vi "报告存储.vi"(8 "生成报告?":bool, 9 "是否存储到数据库?":bool, 11 "试验时间":timestamp) -> ()   [LabVIEW 2010]
uses:
  <vilib>/Utility/NIReport.llb/NI_report.lvclass
  全局量/试验配置信息.vi
  全局量/自动测试结果.vi
  <vilib>/Utility/NIReport.llb/Append Report Text (str wrap).vi
  全局量/全局_配置.vi
  <vilib>/addons/_office/word.llb/Word Easy Table (str).vi
  <vilib>/addons/_office/NI_ReportGenerationToolkit.lvlib
panel:
  in  "序号 2":i32
  in  "序号":i32
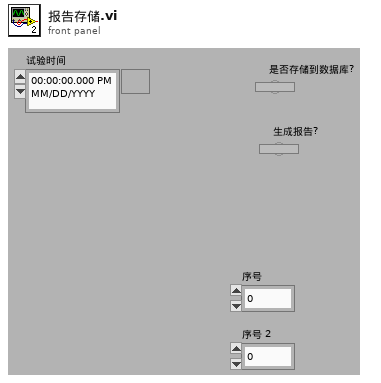
[diagram p1: front panel]
types:
  T1 = enum16{"maximized", "minimized", "normal", "no change"}
  T2 = enum16{"Standard Report", "HTML", "Word", "Excel"}
  T3 = cluster{"position (Excel)":cluster{"row":i32, "column":i32}, "name (Excel)":string, "bookmark (Word)":string}
  T4 = cluster{"报告编号":string, "控制板编号":string, "控制板类型":string, "测试人员":string, "测试地点":string, string, u64, "spreadsheet string":string, "spreadsheet string":string, "spreadsheet string":string, "spreadsheet string":string, "格式字符串":string}
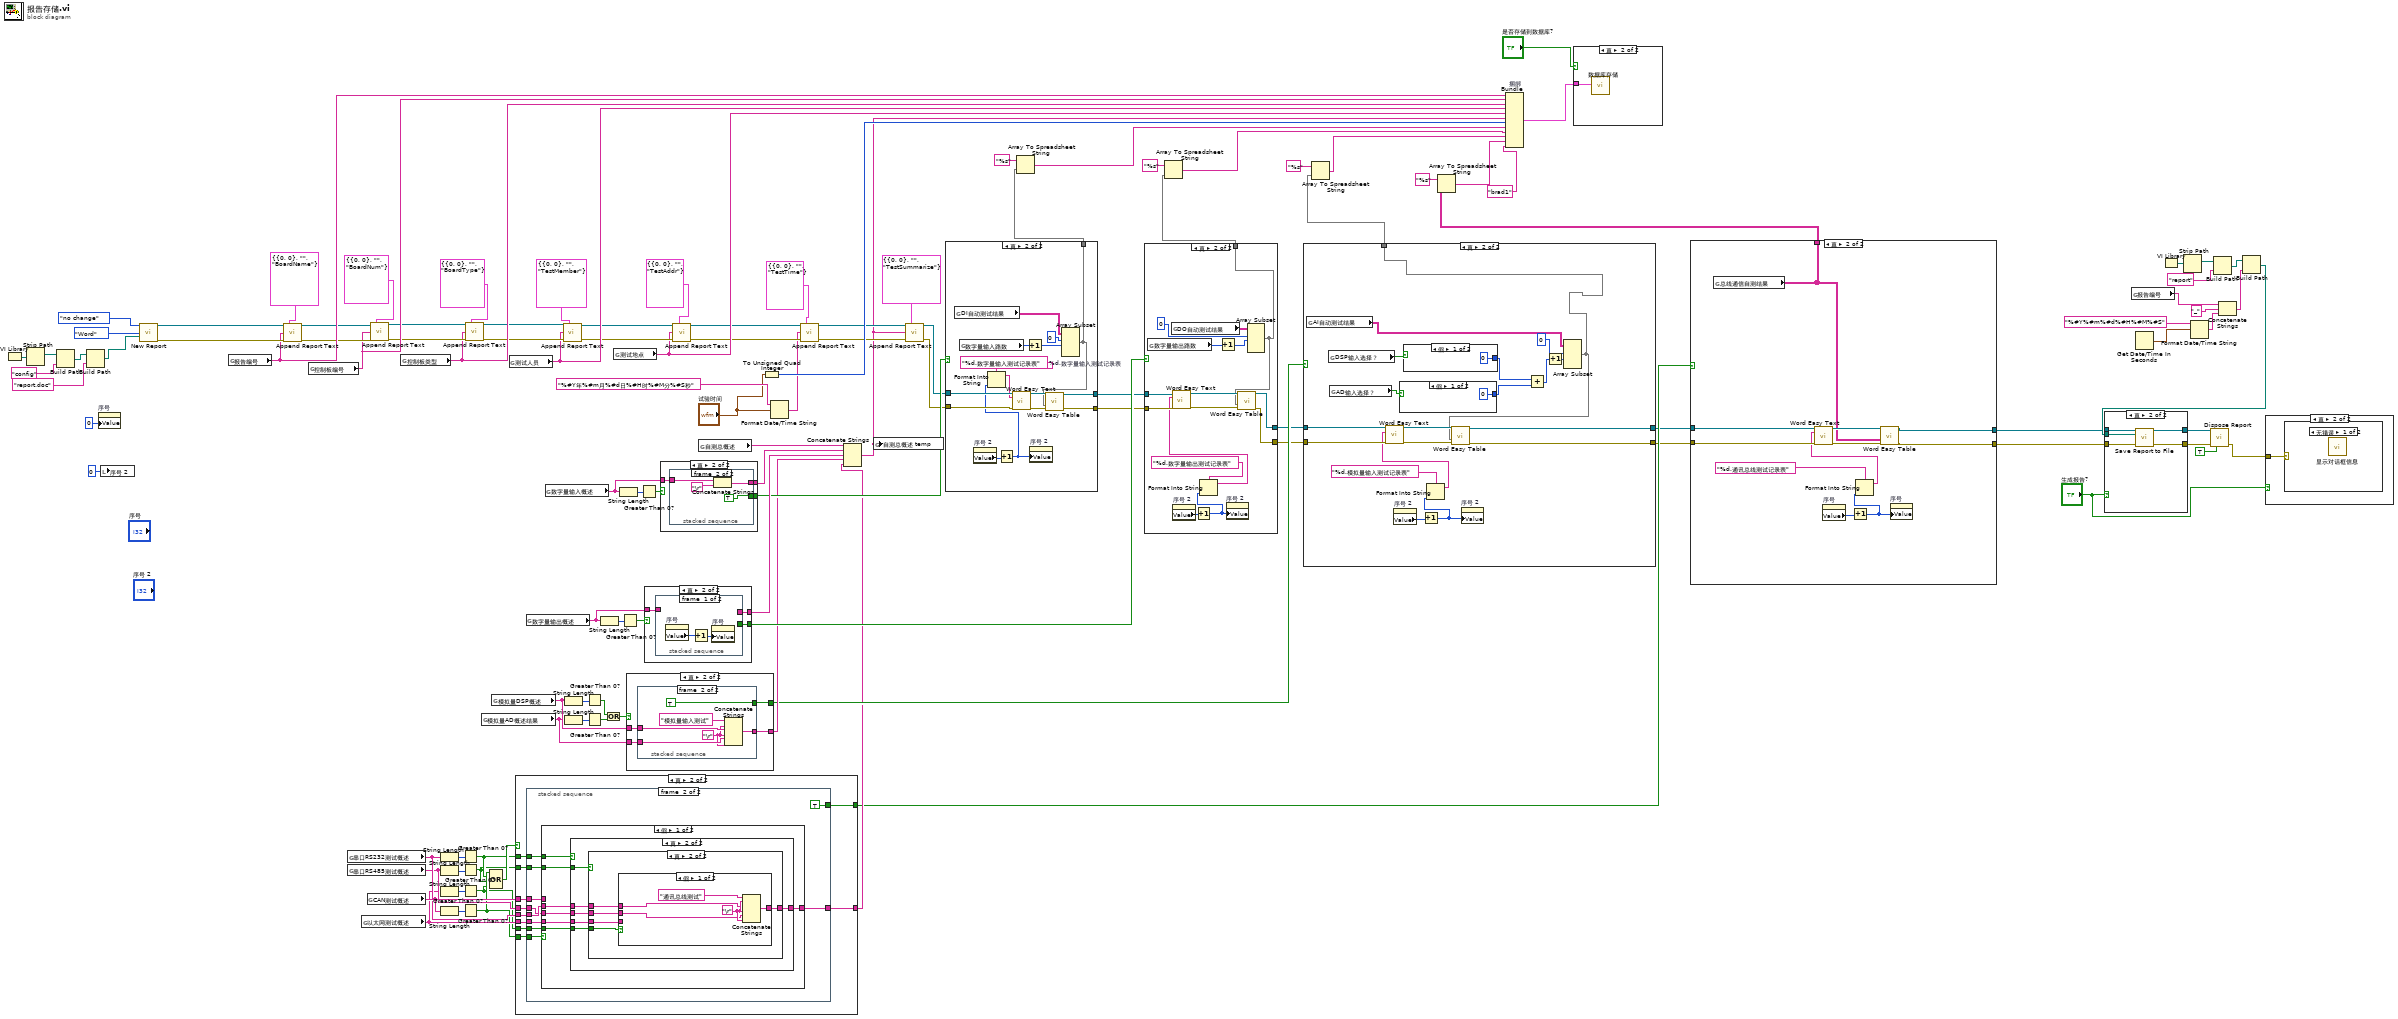
[diagram p0: block diagram]
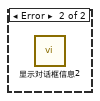
[diagram p3: hidden frame]
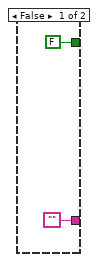
[diagram p6: hidden frame]
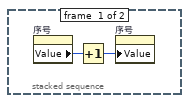
[diagram p7: hidden frame]
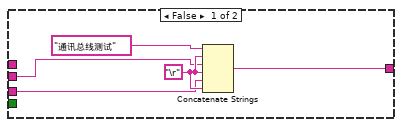
[diagram p8: hidden frame]
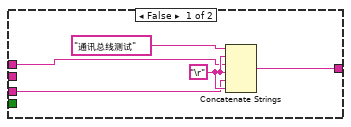
[diagram p9: hidden frame]
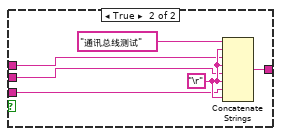
[diagram p10: hidden frame]
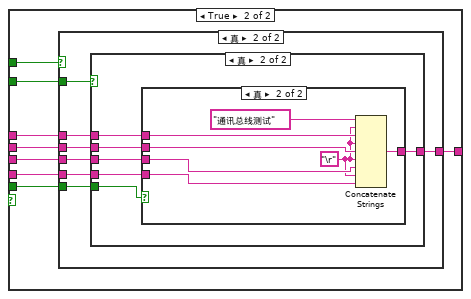
[diagram p11: hidden frame]
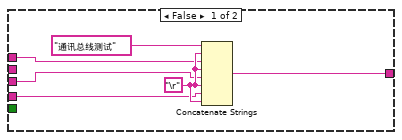
[diagram p12: hidden frame]
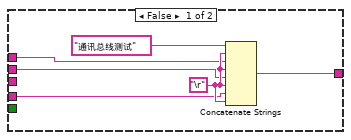
[diagram p13: hidden frame]
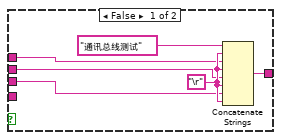
[diagram p14: hidden frame]
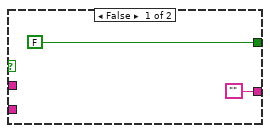
[diagram p15: hidden frame]
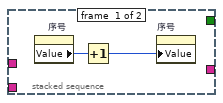
[diagram p16: hidden frame]
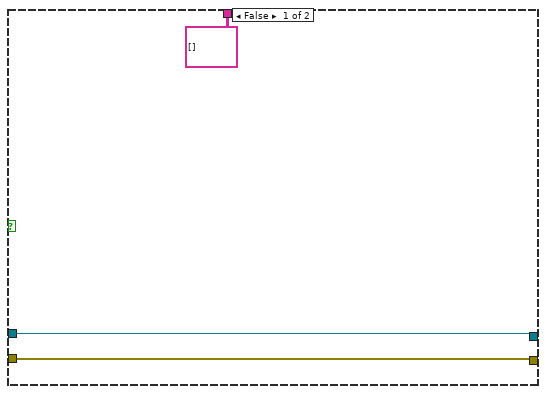
[diagram p17: hidden frame]
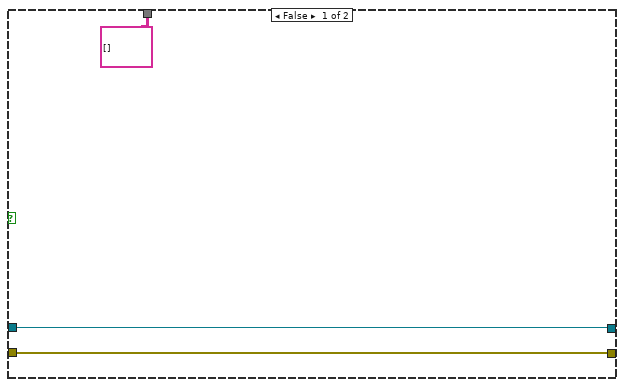
[diagram p18: hidden frame]
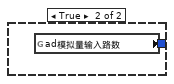
[diagram p19: hidden frame]
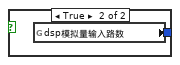
[diagram p20: hidden frame]
diagram:
  n1 = VI Library() -> (path=w67:path)
  n2 = Strip Path(path=w67) -> (stripped path=w64:path)  [unwired: 1 out]
  n3 = Build Path(base path=w64, name or relative path="config") -> (appended path=w66:path)
  n4 = Build Path(base path=w66, name or relative path="report.doc") -> (appended path=w70:path)
  n5 = property on="序号" class="DigNum (严格)"("Value"=0 ("序号")) -> ()  [unwired: 2 in, 2 out]
  n6 = local write "序号 2"(0 ("序号 2")) -> ()
  n7 = call <vilib>:"New Report.vi"("window state (normal)"=T1."no change", "report type"=T2."Word", "template (empty)"=w70) -> ("report out"=w62:refnum<class "NI_report.lvclass">, "error out"=w61:errorcluster)  [unwired: 11 in]
  n8 = global read "试验配置信息.vi" "报告编号"() -> (w60:string)
  n9 = call-poly <vilib>:"Append Report Text.vi"("report in"=w62, "MS Office parameters"=T3 {"position (Excel)"={"row"=0, "column"=0}, "name (Excel)"="", "bookmark (Word)"="BoardName"}, "text"=w60, "error in (no error)"=w61) -> ("report out"=w58:refnum<class "NI_report.lvclass">, "error out"=w57:errorcluster)  [unwired: 8 in, 2 out]
  n10 = global read "试验配置信息.vi" "控制板编号"() -> (w56:string)
  n11 = global read "自动测试结果.vi" "串口RS232测试概述"() -> (w76:string)
  n12 = global read "自动测试结果.vi" "串口RS485测试概述"() -> (w75:string)
  n13 = global read "自动测试结果.vi" "以太网测试概述"() -> (w74:string)
  n14 = global read "自动测试结果.vi" "CAN测试概述"() -> (w77:string)
  n15 = call-poly <vilib>:"Append Report Text.vi"("report in"=w58, "MS Office parameters"=T3 {"position (Excel)"={"row"=0, "column"=0}, "name (Excel)"="", "bookmark (Word)"="BoardNum"}, "text"=w56, "error in (no error)"=w57) -> ("report out"=w54:refnum<class "NI_report.lvclass">, "error out"=w53:errorcluster)  [unwired: 8 in, 2 out]
  n16 = global read "试验配置信息.vi" "控制板类型"() -> (w52:string)
  n17 = String Length(string=w76) -> (length=w80:i32)
  n18 = String Length(string=w75) -> (length=w81:i32)
  n19 = String Length(string=w74) -> (length=w82:i32)
  n20 = String Length(string=w77) -> (length=w79:i32)
  n21 = Greater Than 0?(x=w80) -> (x > 0?=w4:bool)
  n22 = Greater Than 0?(x=w81) -> (x > 0?=w3:bool)
  n23 = Greater Than 0?(x=w82) -> (x > 0?=w2:bool)
  n24 = Greater Than 0?(x=w79) -> (x > 0?=w5:bool)
  n25 = call-poly <vilib>:"Append Report Text.vi"("report in"=w54, "MS Office parameters"=T3 {"position (Excel)"={"row"=0, "column"=0}, "name (Excel)"="", "bookmark (Word)"="BoardType"}, "text"=w52, "error in (no error)"=w53) -> ("report out"=w50:refnum<class "NI_report.lvclass">, "error out"=w49:errorcluster)  [unwired: 8 in, 2 out]
  n26 = global read "自动测试结果.vi" "模拟量AD概述结果"() -> (w85:string)
  n27 = Compound Arithmetic op=OR(w5, w4, w3, w2) -> (w78:bool)
  n28 = global read "自动测试结果.vi" "模拟量DSP概述"() -> (w86:string)
  n29 = global read "试验配置信息.vi" "测试人员"() -> (w48:string)
  n30 = case shown="真" w78 {
    tunnel: ["" w125] -> w73
    tunnel: [FALSE w124] -> w72
    tunnel: w77 -> [_ w129]
    tunnel: w76 -> [_ w128]
    tunnel: w75 -> [_ w127]
    tunnel: w74 -> [_ w126]
    tunnel: w5 -> [_ w123]
    tunnel: w4 -> [_ w122]
    tunnel: w3 -> [_ w121]
    tunnel: w2 -> [_ w120]
    frame False {
    }
    frame True {
      n31 = stacked-sequence {
        tunnel: w129 -> [_ w141]
        tunnel: w128 -> [_ w140]
        tunnel: w127 -> [_ w139]
        tunnel: w126 -> [_ w138]
        tunnel: [_ w137] -> w125
        tunnel: [_ TRUE] -> w124
        tunnel: w123 -> [_ w135]
        tunnel: w122 -> [_ w134]
        tunnel: w121 -> [_ w133]
        tunnel: w120 -> [_ w132]
        frame #0 {
          n32 = property on="序号" class="DigNum (严格)"() -> ("Value"=w130:i32)  [unwired: 2 in, 2 out]
          n33 = Increment(x=w130) -> (x+1=w131:i32)
          n34 = property on="序号" class="DigNum (严格)"("Value"=w131) -> ()  [unwired: 2 in, 2 out]
        }
        frame #1 {
          n35 = case shown="假" w135 {
            tunnel: w141 -> [_ w188]
            tunnel: w140 -> [w147 w187]
            tunnel: w139 -> [w146 w186]
            tunnel: w138 -> [w145 w185]
            tunnel: [w148 w184] -> w137
            tunnel: w134 -> [w144 w183]
            tunnel: w133 -> [w143 w182]
            tunnel: w132 -> [w142 w181]
            frame False {
              n36 = case shown="真" w144 {
                tunnel: [w149 w159] -> w148
                tunnel: w147 -> [_ w158]
                tunnel: w146 -> [w151 w157]
                tunnel: w145 -> [w150 w156]
                tunnel: w143 -> [_ w155]
                tunnel: w142 -> [_ w154]
                frame False {
                  w152 = "\r"
                  n37 = Concatenate Strings("通讯总线测试", w152, w151, w152, w150, w152) -> (w149:string)
                }
                frame True {
                  n38 = case shown="真" w155 {
                    tunnel: [w162 w169] -> w159
                    tunnel: w158 -> [w161 w168]
                    tunnel: w157 -> [_ w167]
                    tunnel: w156 -> [w160 w166]
                    tunnel: w154 -> [_ w165]
                    frame False {
                      w163 = "\r"
                      n39 = Concatenate Strings("通讯总线测试", w163, w161, w163, w160, w163) -> (w162:string)
                    }
                    frame True {
                      n40 = case shown="假" w165 {
                        tunnel: [w172 w178] -> w169
                        tunnel: w168 -> [w171 w177]
                        tunnel: w167 -> [w170 w176]
                        tunnel: w166 -> [_ w175]
                        frame False {
                          w173 = "\r"
                          n41 = Concatenate Strings("通讯总线测试", w173, w171, w173, w170, w173) -> (w172:string)
                        }
                        frame True {
                          w179 = "\r"
                          n42 = Concatenate Strings("通讯总线测试", w179, w177, w179, w176, w179, w175, w179) -> (w178:string)
                        }
                      }
                    }
                  }
                }
              }
            }
            frame True {
              n43 = case shown="真" w183 {
                tunnel: w188 -> [w191 w201]
                tunnel: w187 -> [_ w200]
                tunnel: w186 -> [w190 w199]
                tunnel: w185 -> [w189 w198]
                tunnel: [w192 w197] -> w184
                tunnel: w182 -> [_ w196]
                tunnel: w181 -> [_ w195]
                frame False {
                  w194 = "\r"
                  n44 = Concatenate Strings("通讯总线测试", w194, w191, w194, w190, w194, w189, w194) -> (w192:string)
                }
                frame True {
                  n45 = case shown="真" w196 {
                    tunnel: w201 -> [w204 w213]
                    tunnel: w200 -> [w203 w212]
                    tunnel: w199 -> [_ w211]
                    tunnel: w198 -> [w202 w210]
                    tunnel: [w205 w209] -> w197
                    tunnel: w195 -> [_ w208]
                    frame False {
                      w206 = "\r"
                      n46 = Concatenate Strings("通讯总线测试", w206, w204, w206, w203, w206, w202, w206) -> (w205:string)
                    }
                    frame True {
                      n47 = case shown="真" w208 {
                        tunnel: w213 -> [w216 w225]
                        tunnel: w212 -> [w215 w224]
                        tunnel: w211 -> [w214 w223]
                        tunnel: w210 -> [_ w222]
                        tunnel: [w218 w220] -> w209
                        frame False {
                          w217 = "\r"
                          n48 = Concatenate Strings("通讯总线测试", w217, w216, w217, w215, w217, w214, w217) -> (w218:string)
                        }
                        frame True {
                          w221 = "\r"
                          n49 = Concatenate Strings("通讯总线测试", w221, w225, w221, w224, w221, w223, w221, w222) -> (w220:string)
                        }
                      }
                    }
                  }
                }
              }
            }
          }
        }
      }
    }
  }
  n50 = global read "自动测试结果.vi" "数字量输出概述"() -> (w114:string)
  n51 = global read "自动测试结果.vi" "数字量输入概述"() -> (w115:string)
  n52 = call-poly <vilib>:"Append Report Text.vi"("report in"=w50, "MS Office parameters"=T3 {"position (Excel)"={"row"=0, "column"=0}, "name (Excel)"="", "bookmark (Word)"="TestMember"}, "text"=w48, "error in (no error)"=w49) -> ("report out"=w45:refnum<class "NI_report.lvclass">, "error out"=w44:errorcluster)  [unwired: 8 in, 2 out]
  n53 = String Length(string=w86) -> (length=w90:i32)
  n54 = String Length(string=w85) -> (length=w88:i32)
  n55 = Greater Than 0?(x=w90) -> (x > 0?=w89:bool)
  n56 = Greater Than 0?(x=w88) -> (x > 0?=w87:bool)
  n57 = String Length(string=w114) -> (length=w112:i32)
  n58 = Or(x=w89, y=w87) -> (x .or. y?=w91:bool)
  n59 = global read "试验配置信息.vi" "测试地点"() -> (w43:string)
  n60 = String Length(string=w115) -> (length=w117:i32)
  n61 = Greater Than 0?(x=w112) -> (x > 0?=w113:bool)
  n62 = case shown="真" w91 {
    tunnel: ["" w230] -> w84
    tunnel: w86 -> [_ w232]
    tunnel: w85 -> [_ w231]
    tunnel: [FALSE w229] -> w83
    frame False {
    }
    frame True {
      n63 = stacked-sequence {
        tunnel: w232 -> [_ w240]
        tunnel: w231 -> [_ w239]
        tunnel: [_ w238] -> w230
        tunnel: [_ TRUE] -> w229
        frame #0 {
          n64 = property on="序号" class="DigNum (严格)"() -> ("Value"=w234:i32)  [unwired: 2 in, 2 out]
          n65 = Increment(x=w234) -> (x+1=w233:i32)
          n66 = property on="序号" class="DigNum (严格)"("Value"=w233) -> ()  [unwired: 2 in, 2 out]
        }
        frame #1 {
          w236 = "\r"
          n67 = Concatenate Strings("模拟量输入测试", w236, w240, w236, w239, w236) -> (w238:string)
        }
      }
    }
  }
  n68 = Greater Than 0?(x=w117) -> (x > 0?=w116:bool)
  n69 = case shown="真" w113 {
    tunnel: w114 -> [_ w245]
    tunnel: ["" w244] -> w109
    tunnel: [FALSE w243] -> w106
    frame False {
    }
    frame True {
      n70 = stacked-sequence {
        tunnel: w245 -> [_ w251]
        tunnel: [_ w249] -> w244
        tunnel: [_ TRUE] -> w243
        frame #0 {
          n71 = property on="序号" class="DigNum (严格)"() -> ("Value"=w247:i32)  [unwired: 2 in, 2 out]
          n72 = Increment(x=w247) -> (x+1=w246:i32)
          n73 = property on="序号" class="DigNum (严格)"("Value"=w246) -> ()  [unwired: 2 in, 2 out]
        }
        frame #1 {
          n74 = Concatenate Strings(w251, "\r") -> (w249:string)
        }
      }
    }
  }
  n75 = case shown="真" w116 {
    tunnel: w115 -> [_ w256]
    tunnel: ["" w255] -> w110
    tunnel: [FALSE w254] -> w107
    frame False {
    }
    frame True {
      n76 = stacked-sequence {
        tunnel: w256 -> [_ w262]
        tunnel: [_ w260] -> w255
        tunnel: [_ TRUE] -> w254
        frame #0 {
          n77 = property on="序号" class="DigNum (严格)"() -> ("Value"=w257:i32)  [unwired: 2 in, 2 out]
          n78 = Increment(x=w257) -> (x+1=w258:i32)
          n79 = property on="序号" class="DigNum (严格)"("Value"=w258) -> ()  [unwired: 2 in, 2 out]
        }
        frame #1 {
          n80 = Concatenate Strings(w262, "\r") -> (w260:string)
        }
      }
    }
  }
  n81 = call-poly <vilib>:"Append Report Text.vi"("report in"=w45, "MS Office parameters"=T3 {"position (Excel)"={"row"=0, "column"=0}, "name (Excel)"="", "bookmark (Word)"="TestAddr"}, "text"=w43, "error in (no error)"=w44) -> ("report out"=w41:refnum<class "NI_report.lvclass">, "error out"=w40:errorcluster)  [unwired: 8 in, 2 out]
  n82 = global read "自动测试结果.vi" "自测总概述"() -> (w111:string)
  n83 = To Unsigned Quad Integer(1:"试验时间") -> (0:w105:u64)
  n84 = Format Date/Time String(time format string (%c)="%#Y年%#m月%#d日%#H时%#M分%#S秒" ("时间格式字符串(%c)"), seconds (now)="试验时间") -> (date/time string=w37:string)  [unwired: 1 in]
  n85 = call-poly <vilib>:"Append Report Text.vi"("report in"=w41, "MS Office parameters"=T3 {"position (Excel)"={"row"=0, "column"=0}, "name (Excel)"="", "bookmark (Word)"="TestTime"}, "text"=w37, "error in (no error)"=w40) -> ("report out"=w36:refnum<class "NI_report.lvclass">, "error out"=w35:errorcluster)  [unwired: 8 in, 2 out]
  n86 = Concatenate Strings(w111, w110, w109, w84, w73) -> (w33:string)
  n87 = global write "自动测试结果.vi" "自测总概述 temp"(w33) -> ()
  n88 = call-poly <vilib>:"Append Report Text.vi"("report in"=w36, "MS Office parameters"=T3 {"position (Excel)"={"row"=0, "column"=0}, "name (Excel)"="", "bookmark (Word)"="TestSummarize"}, "text"=w33, "error in (no error)"=w35) -> ("report out"=w32:refnum<class "NI_report.lvclass">, "error out"=w31:errorcluster)  [unwired: 8 in, 2 out]
  n89 = case shown="真" w107 {
    tunnel: [string[][] [] ("DI自动测试结果") w270] -> w103
    tunnel: w32 -> [w264 w276]
    tunnel: w31 -> [w263 w275]
    tunnel: [w264 w267] -> w30
    tunnel: [w263 w266] -> w29
    frame False {
    }
    frame True {
      w272 = "%d.数字量输入测试记录表"  # %d.数字量输入测试记录表
      n90 = global read "自动测试结果.vi" "DI自动测试结果"() -> (w279:string[][])
      n91 = global read "全局_配置.vi" "数字量输入路数"() -> (w278:i32)
      n92 = property on="序号 2" class="DigNum (严格)"() -> ("Value"=w269:i32)  [unwired: 2 in, 2 out]
      n93 = Increment(x=w269) -> (x+1=w268:i32)
      n94 = Format Into String(format string=w272, w268) -> (resulting string=w271:string)  [unwired: 2 in, 1 out]
      n95 = call <vilib>:"Word Easy Text.vi"("report in"=w276, "text"=w271, "error in (no error)"=w275) -> ("report out"=w274:refnum<class "NI_report.lvclass">, "error out"=w273:errorcluster)  [unwired: 10 in, 1 out]
      n96 = Increment(x=w278) -> (x+1=w277:i32)
      n97 = property on="序号 2" class="DigNum (严格)"("Value"=w268) -> ()  [unwired: 2 in, 2 out]
      n98 = Array Subset(array=w279, index (row)=0 ("索引"), length (row)=w277) -> (w270:string[][])  [unwired: 2 in]
      n99 = call-poly <vilib>:"Word Easy Table.vi"("report in"=w274, "data"=w270, "error in (no error)"=w273) -> ("report out"=w267:refnum<class "NI_report.lvclass">, "error out"=w266:errorcluster)  [unwired: 10 in, 1 out]
    }
  }
  n100 = Array To Spreadsheet String(array=w103, 3:"%s" ("格式字符串")) -> (spreadsheet string=w102:string)  [unwired: 1 in]
  n101 = case shown="真" w106 {
    tunnel: [string[][] [] ("DO自动测试结果") w286] -> w100
    tunnel: w30 -> [w282 w291]
    tunnel: w29 -> [w281 w290]
    tunnel: [w282 w285] -> w28
    tunnel: [w281 w284] -> w27
    frame False {
    }
    frame True {
      n102 = global read "全局_配置.vi" "数字量输出路数"() -> (w298:i32)
      n103 = global read "自动测试结果.vi" "DO自动测试结果"() -> (w297:string[][])
      n104 = property on="序号 2" class="DigNum (严格)"() -> ("Value"=w294:i32)  [unwired: 2 in, 2 out]
      n105 = Increment(x=w294) -> (x+1=w293:i32)
      n106 = Format Into String(format string="%d.数字量输出测试记录表", w293) -> (resulting string=w287:string)  [unwired: 2 in, 1 out]
      n107 = call <vilib>:"Word Easy Text.vi"("report in"=w291, "text"=w287, "error in (no error)"=w290) -> ("report out"=w289:refnum<class "NI_report.lvclass">, "error out"=w288:errorcluster)  [unwired: 10 in, 1 out]
      n108 = Increment(x=w298) -> (x+1=w296:i32)
      n109 = property on="序号 2" class="DigNum (严格)"("Value"=w293) -> ()  [unwired: 2 in, 2 out]
      n110 = Array Subset(array=w297, index (row)=0 ("索引"), length (row)=w296) -> (w286:string[][])  [unwired: 2 in]
      n111 = call-poly <vilib>:"Word Easy Table.vi"("report in"=w289, "data"=w286, "error in (no error)"=w288) -> ("report out"=w285:refnum<class "NI_report.lvclass">, "error out"=w284:errorcluster)  [unwired: 10 in, 1 out]
    }
  }
  n112 = Array To Spreadsheet String(array=w100, 3:"%s" ("格式字符串")) -> (spreadsheet string=w99:string)  [unwired: 1 in]
  n113 = case shown="真" w83 {
    tunnel: [string[][] [] ("AI自动测试结果") w304] -> w97
    tunnel: w28 -> [w300 w309]
    tunnel: w27 -> [w299 w308]
    tunnel: [w300 w303] -> w26
    tunnel: [w299 w302] -> w25
    frame False {
    }
    frame True {
      n114 = global read "自动测试结果.vi" "AI自动测试结果"() -> (w318:string[][])
      n115 = global read "试验配置信息.vi" "DSP输入选择？"() -> (w314:bool)
      n116 = global read "试验配置信息.vi" "AD输入选择？"() -> (w313:bool)
      n117 = property on="序号 2" class="DigNum (严格)"() -> ("Value"=w311:i32)  [unwired: 2 in, 2 out]
      n118 = case shown="假" w313 {
        tunnel: [u32 0 ("ad模拟量输入路数") w322] -> w317
        frame False {
        }
        frame True {
          n119 = global read "全局_配置.vi" "ad模拟量输入路数"() -> (w322:u32)
        }
      }
      n120 = case shown="假" w314 {
        tunnel: [u32 0 ("dsp模拟量输入路数") w324] -> w316
        frame False {
        }
        frame True {
          n121 = global read "全局_配置.vi" "dsp模拟量输入路数"() -> (w324:u32)
        }
      }
      n122 = Increment(x=w311) -> (x+1=w312:i32)
      n123 = Format Into String(format string="%d.模拟量输入测试记录表", w312) -> (resulting string=w305:string)  [unwired: 2 in, 1 out]
      n124 = call <vilib>:"Word Easy Text.vi"("report in"=w309, "text"=w305, "error in (no error)"=w308) -> ("report out"=w307:refnum<class "NI_report.lvclass">, "error out"=w306:errorcluster)  [unwired: 10 in, 1 out]
      n125 = property on="序号 2" class="DigNum (严格)"("Value"=w312) -> ()  [unwired: 2 in, 2 out]
      n126 = Add(x=w316, y=w317) -> (x+y=w315:u32)
      n127 = Increment(x=w315) -> (x+1=w319:u32)
      n128 = Array Subset(array=w318, index (row)=0 ("索引 (行)"), length (row)=w319) -> (w304:string[][])  [unwired: 2 in]
      n129 = call-poly <vilib>:"Word Easy Table.vi"("report in"=w307, "data"=w304, "error in (no error)"=w306) -> ("report out"=w303:refnum<class "NI_report.lvclass">, "error out"=w302:errorcluster)  [unwired: 10 in, 1 out]
    }
  }
  n130 = Array To Spreadsheet String(array=w97, 3:"%s" ("格式字符串")) -> (spreadsheet string=w96:string)  [unwired: 1 in]
  n131 = case shown="真" w72 {
    tunnel: [string[][] [] ("总线通信自测结果") w330] -> w94
    tunnel: w26 -> [w326 w334]
    tunnel: w25 -> [w325 w333]
    tunnel: [w326 w329] -> w10
    tunnel: [w325 w328] -> w9
    frame False {
    }
    frame True {
      n132 = global read "自动测试结果.vi" "总线通信自测结果"() -> (w330:string[][])
      n133 = property on="序号" class="DigNum (严格)"() -> ("Value"=w337:i32)  [unwired: 2 in, 2 out]
      n134 = Increment(x=w337) -> (x+1=w336:i32)
      n135 = Format Into String(format string="%d.通讯总线测试记录表", w336) -> (resulting string=w332:string)  [unwired: 2 in, 1 out]
      n136 = call <vilib>:"Word Easy Text.vi"("report in"=w334, "text"=w332, "error in (no error)"=w333) -> ("report out"=w331:refnum<class "NI_report.lvclass">, "error out"=w338:errorcluster)  [unwired: 10 in, 1 out]
      n137 = call-poly <vilib>:"Word Easy Table.vi"("report in"=w331, "data"=w330, "error in (no error)"=w338) -> ("report out"=w329:refnum<class "NI_report.lvclass">, "error out"=w328:errorcluster)  [unwired: 10 in, 1 out]
      n138 = property on="序号" class="DigNum (严格)"("Value"=w336) -> ()  [unwired: 2 in, 2 out]
    }
  }
  n139 = Array To Spreadsheet String(array=w94, 3:"%s" ("格式字符串")) -> (spreadsheet string=w93:string)  [unwired: 1 in]
  n140 = Bundle "捆绑"("报告编号"=w60, "控制板编号"=w56, "控制板类型"=w52, "测试人员"=w48, "测试地点"=w43, w33, w105, "spreadsheet string"=w102, "spreadsheet string"=w99, "spreadsheet string"=w96, "spreadsheet string"=w93, "格式字符串"="brad1") -> (w92:T4)  [unwired: 1 in]
  n141 = case shown="真" "是否存储到数据库?" {
    tunnel: w92 -> [_ w339]
    frame False {
    }
    frame True {
      n142 = call "数据库存储.vi"("输出簇 2"=w339) -> ()  [unwired: 10 in]
    }
  }
  n143 = global read "试验配置信息.vi" "报告编号"() -> (w13:string)
  n144 = Get Date/Time In Seconds() -> (seconds since 1Jan1904=w19:timestamp)
  n145 = VI Library() -> (path=w20:path)
  n146 = Strip Path(path=w20) -> (stripped path=w23:path)  [unwired: 1 out]
  n147 = Format Date/Time String(time format string (%c)="%#Y%#m%#d%#H%#M%#S" ("时间格式字符串(%c)"), seconds (now)=w19) -> (date/time string=w14:string)  [unwired: 1 in]
  n148 = Build Path(base path=w23, name or relative path="report") -> (appended path=w21:path)
  n149 = Concatenate Strings(w13, "_", w14) -> (w11:string)
  n150 = Build Path(base path=w21, name or relative path=w11) -> (appended path=w15:path)
  n151 = case shown="真" "生成报告?" {
    tunnel: w10 -> [w341 w346]
    tunnel: w9 -> [w340 w345]
    tunnel: [w341 w344] -> w17
    tunnel: [w340 w343] -> w16
    tunnel: w15 -> [_ w342]
    frame False {
    }
    frame True {
      n152 = call-dynamic "Save Report to File.vi"("report in"=w346, "report file path"=w342, "error in (no error)"=w345) -> ("report out"=w344:refnum<class "NI_report.lvclass">, "error out"=w343:errorcluster)  [unwired: 11 in]
    }
  }
  n153 = call-dynamic "Dispose Report.vi"("report in"=w17, "error in (no error)"=w16, "close report? (T)"=TRUE) -> ("error out"=w7:errorcluster)  [unwired: 12 in]
  n154 = case shown="真" "生成报告?" {
    tunnel: w7 -> [_ w347]
    frame False {
    }
    frame True {
      n155 = case shown="无错误" w347 {
        frame No Error {
          n156 = call "显示对话框信息"() -> ()  [unwired: 10 in, 2 out]
        }
        frame Error {
          n157 = call "显示对话框信息2"() -> ()  [unwired: 10 in, 2 out]
        }
      }
    }
  }
